vi "single sweep - next chunk - V2.vi"(4 "algorithm":string="statemachine", 6 "mode":enum16{"first time", "uniform", "adaptive"}(ring)=enum."adaptive", 9 "x + iy":cdb[](array[numeric])=[0.0014961444378751654-0.005494848789731022i, 0.0014279223595474386-0.005470747752736027i, 0.001513711413730512-0.00552874878044623i, 0.001502407562898675-0.005445638194888334i, 0.0015845696982058808-0.005437153149732619i, 0.0015101628497750257-0.005522728337901211i, 0.0015131031857027845-0.005520920485579818i, 0.0015751707865244427-0.005432155579139866i, 0.001381283887581937-0.0055376532176146485i, 0.0013869914972504977-0.005471269712968517i], 10 "chunks":T1={"start F (Hz)"=1400000.0, "stop F (Hz)"=3000000.0, "total number of points"=6000, "chunk size"=10, "freq step (Hz)"=400.0, "update rate (Hz)"=250.0, "adaptive parameters"={"peaks are known -- parameters"={"Def Gamma (kHz)"=0.5, "dV"=15.0, "time in Gamma (sec)"=7.0, "phi-star"=0.0, "all peaks (kHz)"=[], "delta t (sec)"=22.0, "default step (Hz)"=0.0, "Max step (Hz)"=0.0, "all gamma (kHz)"=[564.0, 649.0, 987.0, 1133.0, 1214.0, 1585.0, 1763.0, 1823.0, 1880.0, 1899.0, 2032.0, 2138.0, 2221.0, 2270.0, 2350.0, 2456.0, 2580.0, 2634.0, 2831.0, 2960.0, 2965.0, 3131.0, 3328.0, 3469.0, 3553.0, 0.0, 3615.0, 3734.0, 0.0, 0.0, 0.0, 4236.0, 4300.0, 4331.0], "peaks OK"=FALSE, "gamma OK"=FALSE, "near omega (kHz)"=0.0, "near gamma (kHz)"=10000.0}, "find peak - parameters"={"wavepacket"={"R"=0.5, "wave number"=17.0, "delta k"=7.0, "radii vector"=[], "radial section"=[], "wave vector"=22.0, "wavepacket is"=TRUE}, "number of grid points"=70, "decimation threshold"=1, "Voltage range"=0.1, "target freq step"=20.0, "target spot size"=0.05, "factor"=1.0, "another factor"=1.0, "analyze last # sec"=3, "scale factor"=3}}, "total sweep time (sec)"=24.0, "chunk time (sec)"=0.04, "spot size (V)"=5.8152639158694506e-05, "uniform freq step (Hz)"=266.6666666666667, "next start freq (Hz)"=1412960.0000000002} {"next start freq (Hz)" format="%#9_8f"; "uniform freq step (Hz)" format="%#_3f"; "spot size (V)" format="%#_2f"; "adaptive parameters"."find peak - parameters"."wavepacket"."delta k" format="%#_3f"; "adaptive parameters"."find peak - parameters"."wavepacket"."wave number" format="%#_3f"; "adaptive parameters"."find peak - parameters"."wavepacket"."R" format="%#_3f"; "freq step (Hz)" format="%#4_4f"; "stop F (Hz)" format="%#_3f"; "start F (Hz)" format="%#_3f"}, 11 "F Array in":dbl[](array[numeric])=[1408640.0000000002, 1408672.0000000002, 1408704.0000000002, 1408736.0000000002, 1408768.0000000002, 1408800.0000000002, 1408832.0000000002, 1408864.0000000002, 1408896.0000000002, 1408928.0000000002]) -> (1 "fancy circles":cluster{dbl[], dbl[]}[](array[cluster])=[{[0.004347976639836461, 0.0043237329011621035, 0.004251384023380436, 0.004132070991513198, 0.003967675443347089, 0.0037607899948818246, 0.0035146773532270816, 0.00323321886176232, 0.0029208532890330928, 0.002582506826719488, 0.00222351540065057, 0.0018495405200665291, 0.0014664799922359413, 0.001080374910511962, 0.0006973143826813736, 0.0003233395020973332, -3.56519239715844e-05, -0.0003739983862851902, -0.0006863639590144167, -0.0009678224504791784, -0.0012139350921339205, -0.0014208205405991845, -0.001585216088765295, -0.0017045291206325324, -0.0017768779984142003, -0.001801121737088557, -0.0017768779984142003, -0.0017045291206325324, -0.0015852160887652941, -0.001420820540599184, -0.00121393509213392, -0.000967822450479178, -0.0006863639590144162, -0.00037399838628518847, -3.5651923971582664e-05, 0.0003233395020973332, 0.0006973143826813741, 0.0010803749105119625, 0.0014664799922359426, 0.001849540520066531, 0.0022235154006505697, 0.002582506826719488, 0.0029208532890330936, 0.003233218861762321, 0.003514677353227083, 0.0037607899948818254, 0.003967675443347089, 0.004132070991513199, 0.004251384023380437, 0.0043237329011621035], [-0.00253283204245687, -0.0021474888509143563, -0.001768222751695333, -0.0014010149977470693, -0.0010516566747086093, -0.0007256573720308159, -0.00042815829345946126, -0.00016385117718095135, 6.309569569158376e-05, 0.0002491032374014545, 0.0003912379979003752, 0.0004872584271080889, 0.0005356502254961651, 0.0005356502254961651, 0.00048725842710808844, 0.0003912379979003752, 0.00024910323740145405, 6.309569569158376e-05, -0.00016385117718095135, -0.0004281582934594617, -0.0007256573720308154, -0.0010516566747086097, -0.00140101499774707, -0.0017682227516953328, -0.0021474888509143567, -0.002532832042456871, -0.002918175233999384, -0.003297441333218408, -0.003664649087166672, -0.004014007410205131, -0.004340006712882925, -0.004637505791454279, -0.004901812907732789, -0.005128759780605325, -0.005314767322315195, -0.005456902082814115, -0.0055529225120218295, -0.005601314310409906, -0.005601314310409906, -0.005552922512021829, -0.005456902082814115, -0.005314767322315195, -0.0051287597806053235, -0.004901812907732788, -0.004637505791454277, -0.004340006712882922, -0.004014007410205131, -0.0036646490871666704, -0.0032974413332184063, -0.0029181752339993822]}, {[-0.0007985969840225416, -0.0005913945404828922, -0.0003841920969432428, -0.0001769896534035934, 3.0212790136055923e-05, 0.00023741523367570524, 0.0004446176772153548, 0.0006518201207550041, 0.0008590225642946534, 0.0010662250078343027, 0.001273427451373952, 0.0014806298949136016, 0.001687832338453251, 0.0018950347819929002, 0.00210223722553255, 0.0023094396690721986, 0.002516642112611848, 0.0027238445561514977, 0.0029310469996911472, 0.003138249443230796], [-0.004804300169328853, -0.004577153356641655, -0.004350006543954456, -0.004122859731267258, -0.00389571291858006, -0.0036685661058928616, -0.003441419293205663, -0.003214272480518465, -0.0029871256678312666, -0.002759978855144068, -0.00253283204245687, -0.0023056852297696716, -0.002078538417082473, -0.0018513916043952751, -0.0016242447917080766, -0.0013970979790208786, -0.0011699511663336801, -0.0009428043536464817, -0.0007156575409592832, -0.0004885107282720852]}, {[-0.0009980406754980312, -0.0007708938628108329, -0.0005437470501236345, -0.0003166002374364362, -8.945342474923792e-05, 0.00013769338793796033, 0.0003648402006251588, 0.0005919870133123571, 0.0008191338259995553, 0.0010462806386867538, 0.0012734274513739518, 0.0015005742640611503, 0.0017277210767483488, 0.001954867889435547, 0.0021820147021227453, 0.0024091615148099433, 0.002636308327497142, 0.0028634551401843403, 0.0030906019528715387, 0.0033177487655587368], [-0.0004608076070603765, -0.0006680100506000258, -0.0008752124941396752, -0.0010824149376793247, -0.001289617381218974, -0.0014968198247586233, -0.0017040222682982728, -0.0019112247118379222, -0.0021184271553775715, -0.0023256295989172206, -0.00253283204245687, -0.0027400344859965196, -0.002947236929536169, -0.0031544393730758183, -0.003361641816615468, -0.003568844260155117, -0.0037760467036947664, -0.003983249147234416, -0.004190451590774065, -0.004397654034313714]}], 2 "chunks out":T1={"start F (Hz)"=1400000.0, "stop F (Hz)"=3000000.0, "total number of points"=6000, "chunk size"=10, "freq step (Hz)"=400.0, "update rate (Hz)"=250.0, "adaptive parameters"={"peaks are known -- parameters"={"Def Gamma (kHz)"=0.5, "dV"=15.0, "time in Gamma (sec)"=7.0, "phi-star"=0.0, "all peaks (kHz)"=[], "delta t (sec)"=22.0, "default step (Hz)"=0.0, "Max step (Hz)"=0.0, "all gamma (kHz)"=[564.0, 649.0, 987.0, 1133.0, 1214.0, 1585.0, 1763.0, 1823.0, 1880.0, 1899.0, 2032.0, 2138.0, 2221.0, 2270.0, 2350.0, 2456.0, 2580.0, 2634.0, 2831.0, 2960.0, 2965.0, 3131.0, 3328.0, 3469.0, 3553.0, 0.0, 3615.0, 3734.0, 0.0, 0.0, 0.0, 4236.0, 4300.0, 4331.0], "peaks OK"=FALSE, "gamma OK"=FALSE, "near omega (kHz)"=0.0, "near gamma (kHz)"=10000.0}, "find peak - parameters"={"wavepacket"={"R"=0.5, "wave number"=17.0, "delta k"=7.0, "radii vector"=[], "radial section"=[], "wave vector"=22.0, "wavepacket is"=TRUE}, "number of grid points"=70, "decimation threshold"=1, "Voltage range"=0.1, "target freq step"=20.0, "target spot size"=0.05, "factor"=1.0, "another factor"=1.0, "analyze last # sec"=3, "scale factor"=3}}, "total sweep time (sec)"=24.0, "chunk time (sec)"=0.04, "spot size (V)"=5.8152639158694506e-05, "uniform freq step (Hz)"=266.6666666666667, "next start freq (Hz)"=1412960.0000000002} {"next start freq (Hz)" format="%#9_8f"; "uniform freq step (Hz)" format="%#_3f"; "spot size (V)" format="%#_2f"; "adaptive parameters"."find peak - parameters"."wavepacket"."delta k" format="%#_3f"; "adaptive parameters"."find peak - parameters"."wavepacket"."wave number" format="%#_3f"; "adaptive parameters"."find peak - parameters"."wavepacket"."R" format="%#_3f"; "freq step (Hz)" format="%#4_4f"; "stop F (Hz)" format="%#_3f"; "start F (Hz)" format="%#_3f"}, 3 "F Array":dbl[](array[numeric])=[1412960.0000000002, 1413360.0000000002, 1413760.0000000002, 1414160.0000000002, 1414560.0000000002, 1414960.0000000002, 1415360.0000000002, 1415760.0000000002, 1416160.0000000002, 1416560.0000000002])   [LabVIEW 2010]
uses:
  single sweep - frequency chunks.ctl
  single sweep - adaptive parameters.ctl
  next chunk -- parameters.ctl
  find peak -- parameters.ctl
  wavepacket.ctl
  generate wave packet V2.vi
  smart decimate .vi
  set up complex region.vi
  inteference -- find center V2.vi
  find circle corners V3.vi
  draw a line.vi
  draw a circle.vi
  generate linear region.vi
  find circle corners - rescale back.vi
  <vilib>/Analysis/baseanly.llb/Median.vi
  <vilib>/Analysis/baseanly.llb/Mean.vi
panel:
  out "viscosity":dbl
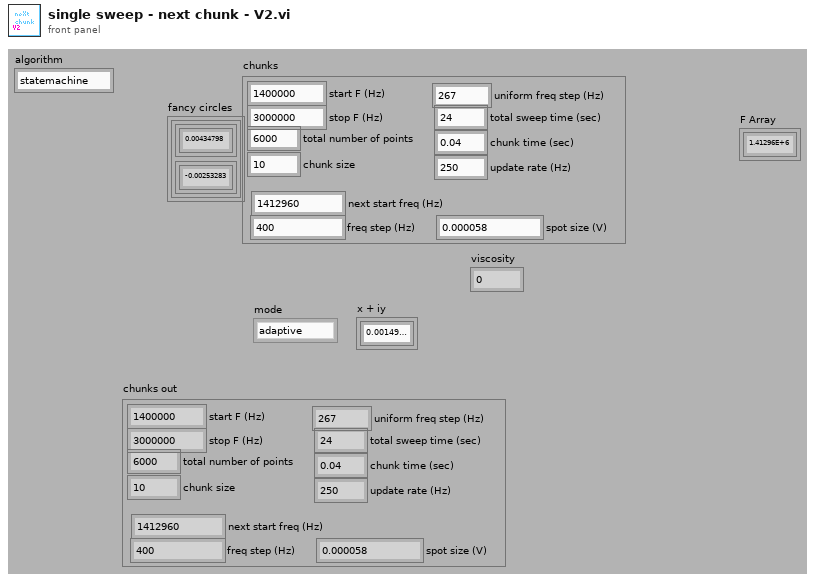
[diagram p1: front panel]
types:
  T1 = typedef "single sweep - frequency chunks.ctl" = cluster{"start F (Hz)":dbl, "stop F (Hz)":dbl, "total number of points":i32, "chunk size":i32, "freq step (Hz)":dbl, "update rate (Hz)":dbl, "adaptive parameters":T2, "total sweep time (sec)":dbl, "chunk time (sec)":dbl, "spot size (V)":dbl, "uniform freq step (Hz)":dbl, "next start freq (Hz)":dbl}
  T2 = typedef "single sweep - adaptive parameters.ctl" = cluster{"peaks are known -- parameters":T3, "find peak - parameters":T4}
  T3 = typedef "next chunk -- parameters.ctl" = cluster{"Def Gamma (kHz)":dbl, "dV":dbl, "time in Gamma (sec)":dbl, "phi-star":dbl, "all peaks (kHz)":dbl[], "delta t (sec)":dbl, "default step (Hz)":dbl, "Max step (Hz)":dbl, "all gamma (kHz)":dbl[], "peaks OK":bool, "gamma OK":bool, "near omega (kHz)":dbl, "near gamma (kHz)":dbl}
  T4 = typedef "find peak -- parameters.ctl" = cluster{"wavepacket":T5, "number of grid points":i32, "decimation threshold":i32, "Voltage range":dbl, "target freq step":dbl, "target spot size":dbl, "factor":dbl, "another factor":dbl, "analyze last # sec":i32, "scale factor":i32}
  T5 = typedef "wavepacket.ctl" = cluster{"R":dbl, "wave number":dbl, "delta k":dbl, "radii vector":dbl[], "radial section":cdb[], "wave vector":dbl, "wavepacket is":bool}
  T6 = typedef "circle corners.ctl" = cluster{"z (-pi/2)":cdb, "z(inf)":cdb, "z (pi/2)":cdb, "z center":cdb, "z(0)":cdb, "radius":dbl}
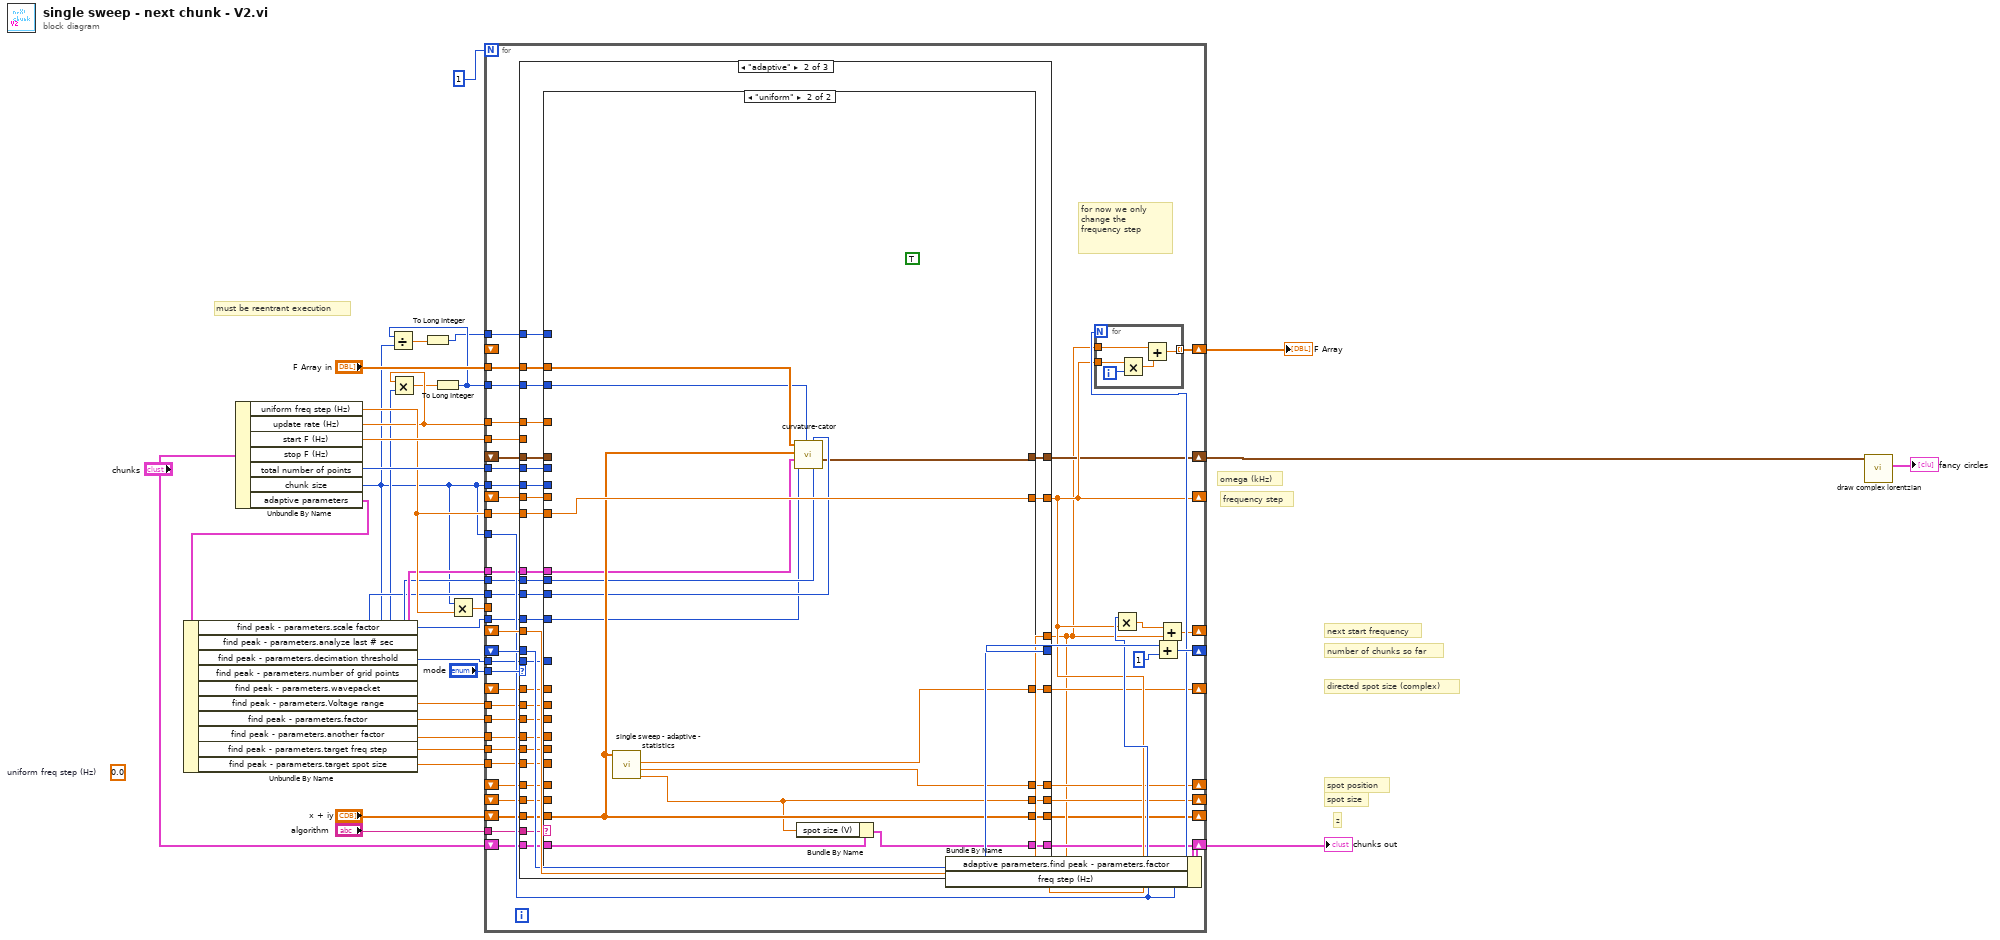
[diagram p0: block diagram]
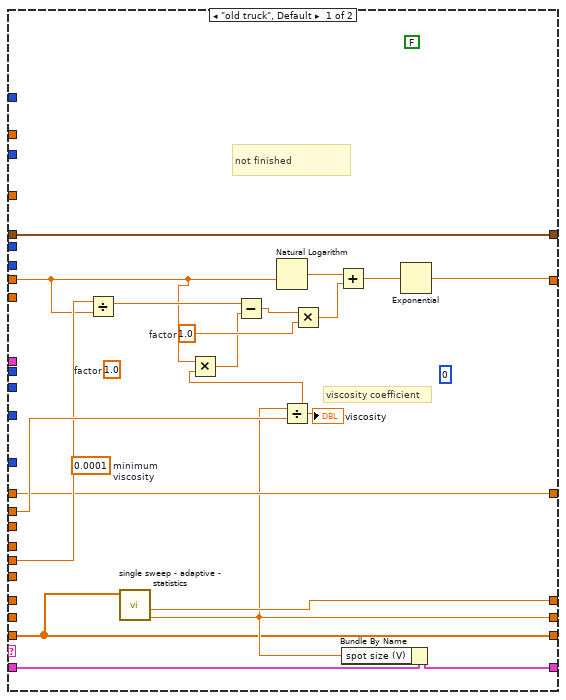
[diagram p3: hidden frame]
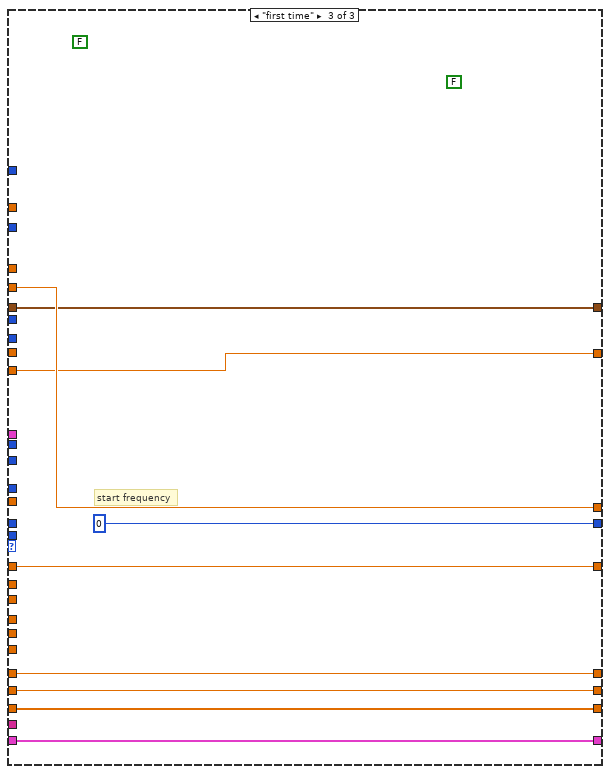
[diagram p4: hidden frame]
diagram:
  (unwired) 0.0  # uniform freq step (Hz)
  # "omega (kHz)"
  # "z"
  # "must be reentrant execution"
  # "directed spot size (complex)"
  # "spot position"
  # "spot size"
  # "frequency step"
  # "number of chunks so far"
  # "next start frequency"
  n1 = Unbundle By Name("chunks") -> ("uniform freq step (Hz)"=w16:dbl, "update rate (Hz)"=w14:dbl, "start F (Hz)"=w29:dbl, "total number of points"=w25:i32, "chunk size"=w6:i32, "adaptive parameters"=w22:T2)  [unwired: 1 out]
  n2 = Unbundle By Name(w22) -> ("find peak - parameters.scale factor"=w1:i32, "find peak - parameters.analyze last # sec"=w10:i32, "find peak - parameters.decimation threshold"=w11:i32, "find peak - parameters.number of grid points"=w12:i32, "find peak - parameters.wavepacket"=w13:T5, "find peak - parameters.Voltage range"=w18:dbl, "find peak - parameters.factor"=w20:dbl, "find peak - parameters.another factor"=w19:dbl, "find peak - parameters.target freq step"=w21:dbl, "find peak - parameters.target spot size"=w17:dbl)
  n3 = Multiply(x=w14, y=w10) -> (x*y=w9:dbl)
  n4 = To Long Integer(number=w9) -> (32bit integer=w7:i32)
  n5 = Divide(x=w7, y=w6) -> (x/y=w5:dbl)
  n6 = To Long Integer(number=w5) -> (32bit integer=w4:i32)
  n7 = Multiply(x=w6, y=w16) -> (x*y=w30:dbl)
  n8 = for {
    N: 1 -> [_]
    tunnel: w16 -> [w46]
    tunnel: w6 -> [w68]
    tunnel: "mode" -> [w76]
    shift-right: [w36] -> _
    shift-left: _ -> [w74]
    shift-right: [w71] -> _
    shift-left: _ -> [w73]
    tunnel: w30 -> [_]
    tunnel: w29 -> [w69]
    shift-right: [w75] -> w8
    shift-left: _ -> [_]
    tunnel: "F Array in" -> [w65]
    tunnel: w6 -> [w64]
    tunnel: w25 -> [w63]
    tunnel: w18 -> [w62]
    shift-right: [w61] -> w24
    shift-left: "chunks" -> [w56]
    shift-right: [w60] -> _
    shift-left: _ -> [w59]
    tunnel: "algorithm" -> [w58]
    tunnel: w21 -> [w57]
    shift-right: [w54] -> _
    shift-left: _ -> [w51]
    shift-right: [w53] -> _
    shift-left: _ -> [w52]
    tunnel: w6 -> [w50]
    shift-right: [w49] -> _
    shift-left: _ -> [w47]
    tunnel: w17 -> [w48]
    tunnel: w20 -> [w45]
    tunnel: w19 -> [w44]
    tunnel: w14 -> [w43]
    tunnel: w7 -> [w42]
    tunnel: w13 -> [w41]
    tunnel: w12 -> [w40]
    tunnel: w11 -> [w39]
    shift-right: [w38] -> w2
    shift-left: _ -> [w37]
    shift-right: [w34] -> _
    shift-left: "x + iy" -> [w66]
    tunnel: w4 -> [w33]
    tunnel: w1 -> [w32]
    # "for now we only change the \nfrequency step"
    n9 = case shown="\"adaptive\"" w76 {
      tunnel: [w85 w119 w160] -> w35
      tunnel: [w83 w118 0] -> w72
      tunnel: w74 -> [w85 w119 _]
      tunnel: w73 -> [w83 w118 _]
      tunnel: w69 -> [_ _ w160]
      tunnel: [w84 w116 w155] -> w60
      tunnel: w59 -> [w84 w117 _]
      tunnel: w66 -> [w77 w115 w153]
      tunnel: w65 -> [_ w114 _]
      tunnel: w64 -> [_ w113 _]
      tunnel: w63 -> [_ w112 _]
      tunnel: w62 -> [_ w111 _]
      tunnel: w58 -> [_ w110 _]
      tunnel: w57 -> [_ w109 _]
      tunnel: w56 -> [w82 w108 w159]
      tunnel: [w82 w107 w159] -> w55
      tunnel: [w80 w106 w157] -> w54
      tunnel: [w81 w105 w158] -> w53
      tunnel: w52 -> [w81 w104 w158]
      tunnel: w51 -> [w80 w103 w157]
      tunnel: w50 -> [_ w102 _]
      tunnel: [w79 w101 w156] -> w49
      tunnel: w48 -> [_ w100 _]
      tunnel: w47 -> [w79 w99 w156]
      tunnel: w46 -> [_ w96 w155]
      tunnel: w45 -> [_ w98 _]
      tunnel: w44 -> [_ w97 _]
      tunnel: w43 -> [_ w95 _]
      tunnel: w42 -> [_ w94 _]
      tunnel: w41 -> [_ w93 _]
      tunnel: w40 -> [_ w92 _]
      tunnel: w39 -> [_ w91 _]
      tunnel: [w78 w90 w154] -> w38
      tunnel: w37 -> [w78 w89 w154]
      tunnel: [w77 w88 w153] -> w34
      tunnel: w33 -> [_ w87 _]
      tunnel: w32 -> [_ w86 _]
      frame "uniform" {
        # "keep frequency step constant,  as determined by global values"
      }
      frame "adaptive" {
        n10 = case shown="\"uniform\"" w110 {
          tunnel: w117 -> [w125 _]
          tunnel: [w128 w152] -> w116
          tunnel: w115 -> [w120 w148]
          tunnel: w114 -> [_ w149]
          tunnel: w113 -> [_ _]
          tunnel: w112 -> [_ _]
          tunnel: w111 -> [w134 _]
          tunnel: w109 -> [w133 _]
          tunnel: w108 -> [w136 w140]
          tunnel: [w135 w141] -> w107
          tunnel: [w122 w142] -> w106
          tunnel: [w123 w151] -> w105
          tunnel: w104 -> [_ _]
          tunnel: w103 -> [_ _]
          tunnel: w102 -> [_ _]
          tunnel: [w124 w150] -> w101
          tunnel: w100 -> [_ _]
          tunnel: w99 -> [w124 _]
          tunnel: w98 -> [_ _]
          tunnel: w97 -> [_ _]
          tunnel: w96 -> [_ w152]
          tunnel: w95 -> [_ _]
          tunnel: w94 -> [_ w144]
          tunnel: w93 -> [_ w147]
          tunnel: w92 -> [_ w145]
          tunnel: w91 -> [_ w146]
          tunnel: [w121 w143] -> w90
          tunnel: w89 -> [w121 _]
          tunnel: [w120 w148] -> w88
          tunnel: w87 -> [_ _]
          tunnel: w86 -> [_ w139]
          frame "old truck", Default {
            (unwired) 0
            (unwired) FALSE
            (unwired) 1.0  # factor
            w131 = 1.0  # factor
            (unwired) 0.0001  # minimum  viscosity
            # "not finished"
            # "viscosity coefficient"
            n11 = Divide(x=w133, y=w125) -> (x/y=w132:dbl)
            n12 = call "single sweep - adaptive - statistics.vi"("x + iy"=w120) -> ("spot size"=w122:dbl, "spot position"=w123:cdb)  [unwired: 8 in, 1 out]
            n13 = Natural Logarithm(1:w125) -> (0:w130:dbl)
            n14 = Divide(x=w122, y=w134) -> (x/y=w127:dbl)
            "viscosity" <- w127
            n15 = Multiply(x=w125, y=w127) -> (x*y=w126:dbl)
            n16 = Subtract(x=w132, y=w126) -> (x-y=w138:dbl)
            n17 = Multiply(x=w138, y=w131) -> (x*y=w137:dbl)
            n18 = Add(x=w130, y=w137) -> (x+y=w129:dbl)
            n19 = Bundle By Name(cluster=w136, "spot size (V)"=w122) -> (w135:T1)
            n20 = Exponential(1:w129) -> (0:w128:dbl)
          }
          frame "uniform" {
            (unwired) TRUE
            n21 = call "single sweep - adaptive - statistics.vi"("x + iy"=w148) -> ("spot size"=w142:dbl, "spot position"=w151:cdb, "spot directed size"=w150:cdb)  [unwired: 8 in]
            n22 = call "curvature-cator.vi"("number of grid points"=w145, "decimation threshold"=w146, "size"=w144, "scale factor"=w139, "wavepacket in"=w147, "z array in"=w148, "omega array in"=w149) -> ("4 corners out"=w143:T6)  [unwired: 2 in, 2 out]
            n23 = Bundle By Name(cluster=w140, "spot size (V)"=w142) -> (w141:T1)
          }
        }
      }
      frame "first time" {
        (unwired) FALSE
        (unwired) FALSE
        # "start frequency"
      }
    }
    n24 = Bundle By Name(cluster=w55, "adaptive parameters.find peak - parameters.factor"=w35, "freq step (Hz)"=w60) -> (w61:T1)
    n25 = for {
      N: w68 -> [_]
      tunnel: w60 -> [w166]
      tunnel: [w164] -> w75 mode=indexing
      tunnel: w35 -> [w162]
      i -> [w163]
      n26 = Multiply(x=w166, y=w163) -> (x*y=w165:dbl)
      n27 = Add(x=w162, y=w165) -> (x+y=w164:dbl)
    }
    n28 = Multiply(x=w68, y=w60) -> (x*y=w67:dbl)
    n29 = Add(x=w72, y=1) -> (x+y=w71:i32)
    n30 = Add(x=w67, y=w35) -> (x+y=w36:dbl)
  }
  "F Array" <- w8
  "chunks out" <- w24
  n31 = call "draw complex lorentzian.vi"("4 corners"=w2) -> ("fancy circles"=→"fancy circles":cluster{dbl[], dbl[]}[])  [unwired: 10 in]
